vi "Write Key Value - Path.vi"(4 "Relative? (F)":bool, 5 "application directory":path, 7 "Value":path, 8 "error in (no error)":errorcluster, 9 "key":string, 10 "section":string, 11 "file refnum in":T1) -> (0 "error out":errorcluster, 3 "file refnum out":T1)   [LabVIEW 2019, in "TSC File IO.lvlib"]
doc: "This VI will write a section/key configuration file of the type:\n<b>Path</b>\n\n<b>Note:</b> The VI will resolve relative paths that will be relative to the input ini file path and the symbolic paths. This gives flexibility to defining key/value pairs for absolute and relative paths.\n\n<appdir> : use the input application directory or the application directory primative (if blank)\n<temp> : the OS temporary directory\n<userdoc> : logged in user's documents folder (Windows)\n<userdesktop> : logged in user's desktop folder (Windows)\n<programdata> : ProgramData folder (Windows)\n<bootdir> : the OS install drive (Windows)\n<programfiles> : the installation directory of applications (Windows)\n..\\ : nomenclature of relative path to the ini file directory\n\nInputs:\n-Path [path] - a path to the file\n-section [string] - the section string in the configuration file\n-key [string] - the key to be read in the configuration file\n-value [Path] - the output data written\n-error in\n\nOutputs:\n-error out\n\n<b>Code Developed By:</b>\nDaniel Coons\nTechnology Service Corporation\n1983 S Liberty Drive\nBloomington, IN 47403\nwww.tsc.com\\atcs"
uses:
  TSC File IO.lvlib
  <vilib>/Utility/config.llb/Config Data RefNum.ctl
  <vilib>/Utility/config.llb/Write Key (Path).vi
  <vilib>/Utility/config.llb/NI_LVConfig.lvlib
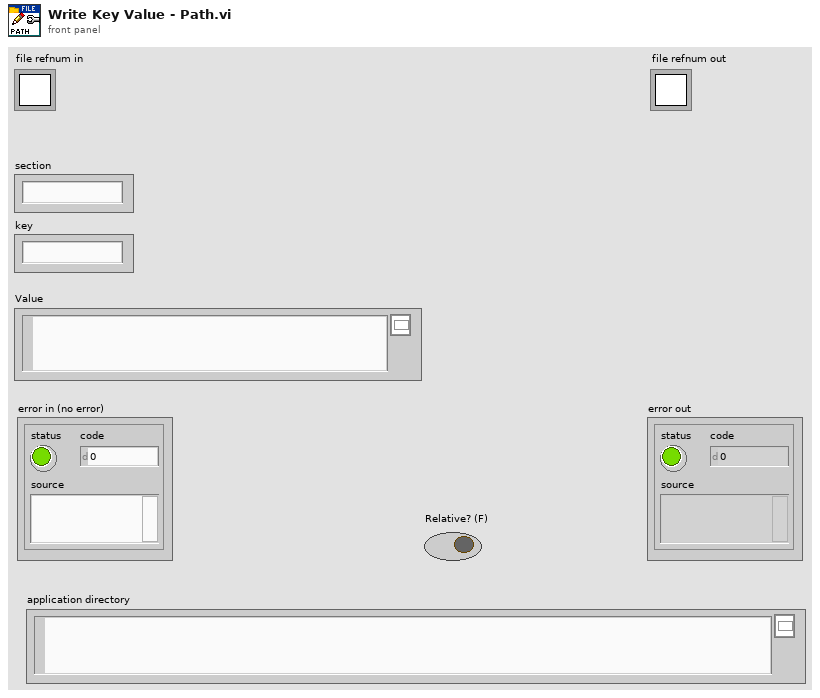
[diagram p1: front panel]
types:
  T1 = typedef "NI_LVConfig.lvlib/Config Data RefNum.ctl" = refnum<k1>
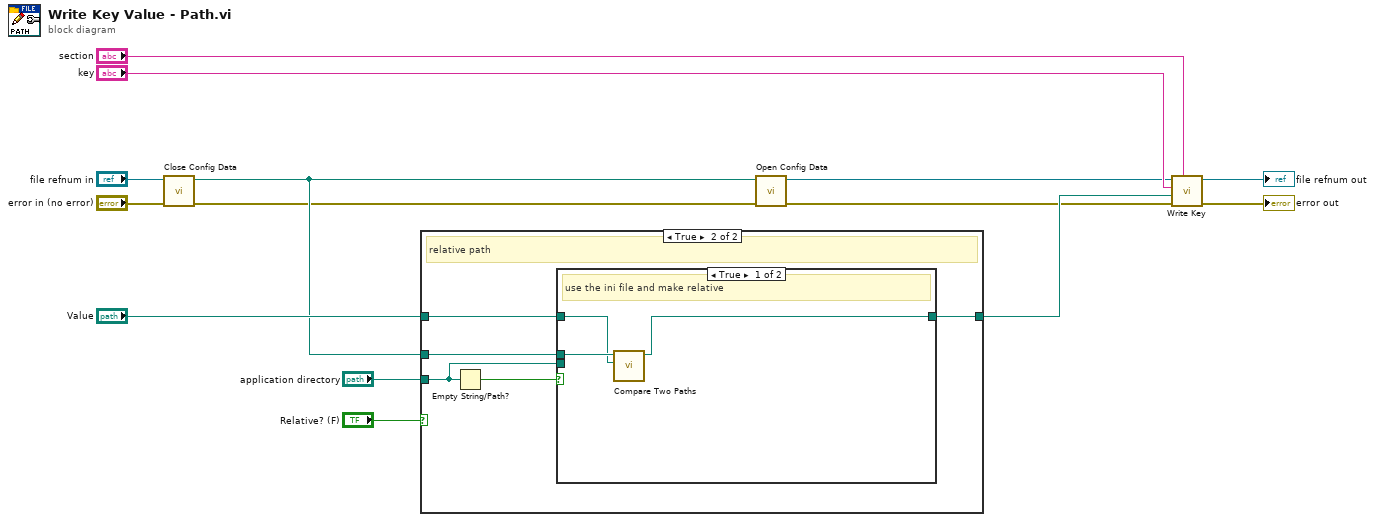
[diagram p0: block diagram]
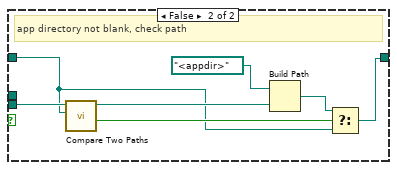
[diagram p3: hidden frame]
diagram:
  n1 = call <vilib>:"Close Config Data.vi"("error in (no error)"="error in (no error)", "refnum"="file refnum in") -> ("error out"=w5:errorcluster, "file path"=w6:path)  [unwired: 8 in]
  n2 = case shown="True" "Relative? (F)" {
    tunnel: "Value" -> [w15 w19]
    tunnel: [w15 w18] -> w9
    tunnel: "application directory" -> [_ w16]
    tunnel: w6 -> [_ w20]
    frame False {
      # "absolute path"
    }
    frame True {
      # "relative path"
      n3 = Empty String/Path?(string/path=w16) -> (empty?=w17:bool)
      n4 = case shown="True" w17 {
        tunnel: w20 -> [w23 _]
        tunnel: w19 -> [w22 w24]
        tunnel: [w21 w25] -> w18
        tunnel: w16 -> [_ w30]
        frame True {
          # "use the ini file and make relative"
          n5 = call <vilib>:"Compare Two Paths.vi"("Path 2"=w22, "Path 1"=w23) -> ("Relative Path from 1 to 2"=w21:path)  [unwired: 6 in, 3 out]
        }
        frame False {
          # "app directory not blank, check path"
          n6 = call <vilib>:"Compare Two Paths.vi"("Path 2"=w24, "Path 1"=w30) -> ("Path 2 Relative to Path 1?"=w27:bool, "Relative Path from 1 to 2"=w28:path)  [unwired: 6 in, 2 out]
          n7 = Build Path(base path=path "<appdir>", name or relative path=w28) -> (appended path=w26:path)
          n8 = Select(t=w26, s=w27, f=w24) -> (s? t:f=w25:path)
        }
      }
    }
  }
  n9 = call <vilib>:"Open Config Data.vi"("error in (no error)"=w5, "configuration file path"=w6) -> ("error out"=w4:errorcluster, "refnum"=w3:T1)  [unwired: 7 in, 1 out]
  n10 = call-poly <vilib>:"Write Key.vi"("section"="section", "error in (no error)"=w4, "value"=w9, "key"="key", "refnum"=w3) -> ("error out"=→"error out":errorcluster, "refnum out"=→"file refnum out":T1)  [unwired: 4 in, 1 out]
